vi "CurrentServoConnectionParameters.vi"(8 "New Servo Connection Parameters":T1={"host"="192.168.0.13", "port"=1, "use_https"=FALSE, "timeout_ms"=5000, "base_url"="http://192.168.0.13:9090"}, 11 "Operation":T2) -> (3 "Current Servo Connection Parameters":T1={"host"="192.168.0.13", "port"=1, "use_https"=FALSE, "timeout_ms"=5000, "base_url"="http://192.168.0.13:9090"})   [LabVIEW 2024]
uses:
  DataTypes/OperationTypeForFunctionalGlobalVariable.ctl
  DataTypes/ServoConnectionParameters.ctl
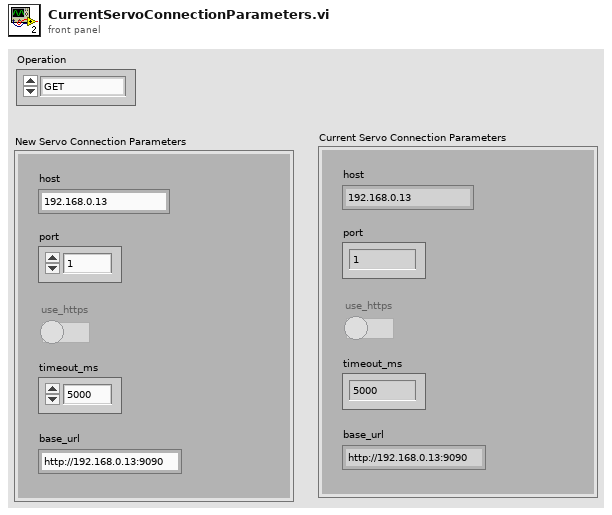
[diagram p1: front panel]
types:
  T1 = typedef "ServoConnectionParameters.ctl" = cluster{"host":string, "port":u16, "use_https":bool, "timeout_ms":u16, "base_url":string}
  T2 = typedef "OperationTypeForFunctionalGlobalVariable.ctl" = enum16{"GET", "SET"}
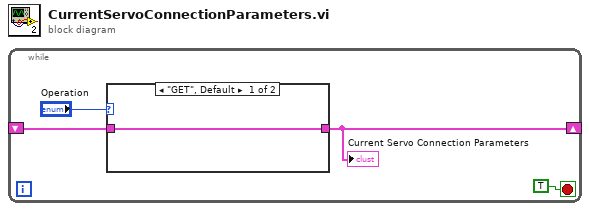
[diagram p0: block diagram]
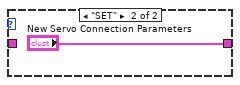
[diagram p2: hidden frame]
diagram:
  n1 = while {
    shift-right: [w1] -> _
    shift-left: _ -> [w3]
    stop <- TRUE stop-if-true
    n2 = case shown="\"GET\", Default" "Operation" {
      tunnel: w3 -> [w5 _]
      tunnel: [w5 "New Servo Connection Parameters"] -> w1
      frame "GET", Default {
      }
      frame "SET" {
      }
    }
    "Current Servo Connection Parameters" <- w1
  }
